vi "FGV_timer.vi"(3 "error in (no error)":errorcluster, 4 "time target":dbl, 5 "action":enum16{"get time", "start timer"}(ring)=enum."start timer") -> (0 "error out":errorcluster, 1 "time elapsed?":bool, 2 "elapsed time":dbl)   [LabVIEW 2019, in "Prueba.lvclass"]
uses:
  Prueba/Prueba.lvclass
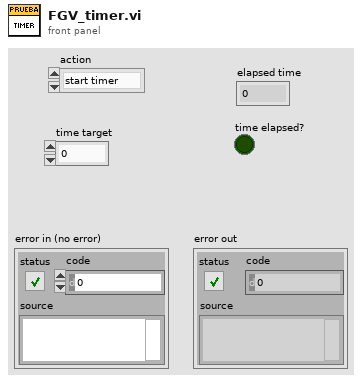
[diagram p1: front panel]
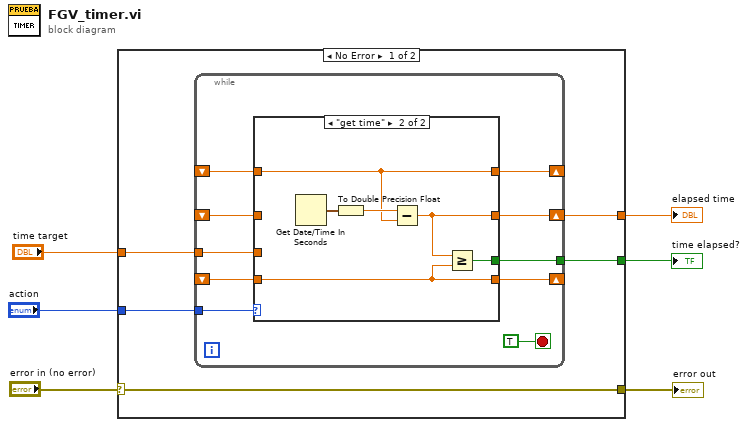
[diagram p0: block diagram]
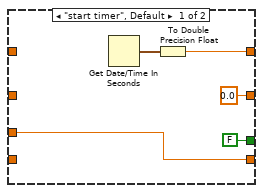
[diagram p2: hidden frame]
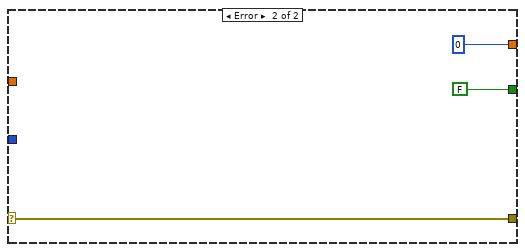
[diagram p3: hidden frame]
diagram:
  n1 = case shown="No Error" "error in (no error)" {
    selector: "error in (no error)" -> [w9 w35]
    tunnel: "action" -> [w11 _]
    tunnel: [w10 0 ("fila_inicial")] -> w5
    tunnel: "time target" -> [w7 _]
    tunnel: [w9 w35] -> w2
    tunnel: [w8 FALSE] -> w1
    frame No Error {
      n2 = while {
        tunnel: w11 -> [w21]
        shift-right: [w20] -> w10
        shift-left: _ -> [w14]
        shift-right: [w17] -> _
        shift-left: _ -> [w16]
        tunnel: [w19] -> w8
        tunnel: w7 -> [w15]
        shift-right: [w13] -> _
        shift-left: _ -> [w12]
        stop <- TRUE stop-if-true
        n3 = case shown="\"get time\"" w21 {
          tunnel: [0.0 ("time target") w30] -> w20
          tunnel: w15 -> [w22 _]
          tunnel: [FALSE w29] -> w19
          tunnel: [w25 w28] -> w17
          tunnel: w16 -> [_ w28]
          tunnel: w14 -> [_ _]
          tunnel: [w22 w27] -> w13
          tunnel: w12 -> [_ w27]
          frame "start timer", Default {
            n4 = Get Date/Time In Seconds() -> (seconds since 1Jan1904=w26:timestamp)
            n5 = To Double Precision Float(number=w26) -> (double precision float=w25:dbl)
          }
          frame "get time" {
            n6 = Get Date/Time In Seconds() -> (seconds since 1Jan1904=w32:timestamp)
            n7 = To Double Precision Float(number=w32) -> (double precision float=w31:dbl)
            n8 = Subtract(x=w31, y=w28) -> (x-y=w30:dbl)
            n9 = Greater Or Equal?(x=w30, y=w27) -> (x >= y?=w29:bool)
          }
        }
      }
    }
    frame Error {
    }
  }
  "elapsed time" <- w5
  "error out" <- w2
  "time elapsed?" <- w1
